vi "to string 1.0.vi"(8 "error in (no error)":errorcluster, 11 "Formatter Config in":refnum<class "csv-formatter Config.lvclass">) -> (0 "error out":errorcluster, 2 "data":string, 3 "Formatter Config out":refnum<class "csv-formatter Config.lvclass">)   [LabVIEW 2015, in "csv-formatter Config.lvclass"]
uses:
  csv-formatter Config.lvclass
  csv-formatter Config.lvclass/csv-formatter Config.ctl
  Result Config.ctl
  <vilib>/NI/Configuration Framework/serializable configuration/NISE_CEF_serializable configuration.lvclass
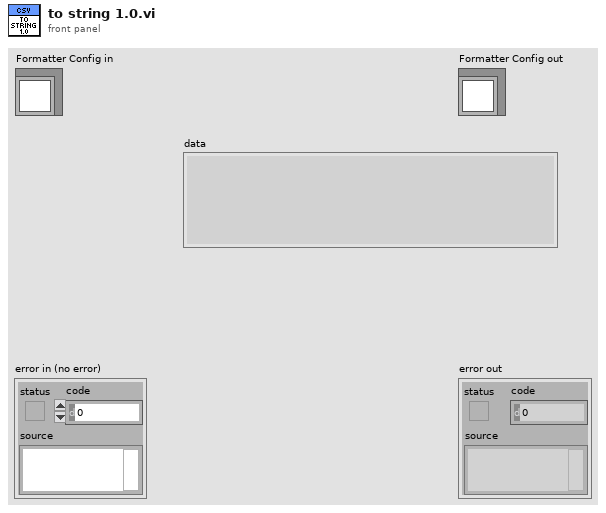
[diagram p1: front panel]
types:
  T1 = typedef "Result Config.ctl" = string[]
  T2 = typedef "Report Header Config.ctl" = string[][]
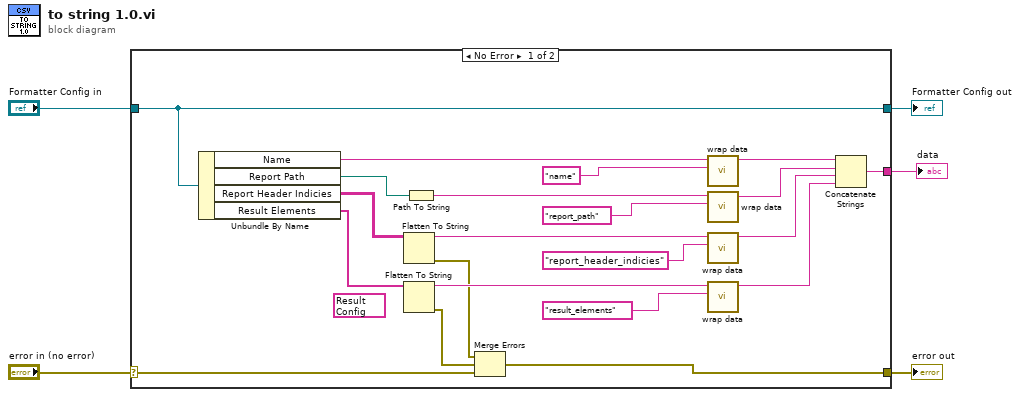
[diagram p0: block diagram]
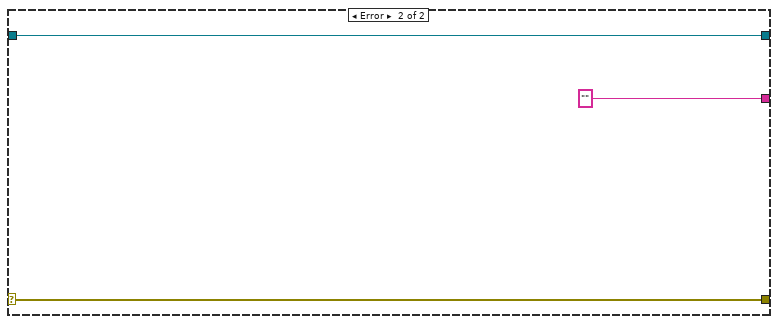
[diagram p2: hidden frame]
diagram:
  n1 = case shown="No Error" "error in (no error)" {
    selector: "error in (no error)" -> [w26 w29]
    tunnel: [w8 w29] -> w4
    tunnel: [w25 w28] -> w2
    tunnel: "Formatter Config in" -> [w25 w28]
    tunnel: [w19 ""] -> w1
    frame No Error {
      (unwired) T1 ["Step Name", "Step Class", "Low Limit", "Measurement", "High Limit", "Comparison", "Duration"] ("Result Elements")
      n2 = Unbundle By Name(w25) -> ("Name"=w23:string, "Report Path"=w22:path, "Report Header Indicies"=w16:T2, "Result Elements"=w12:T1)
      n3 = Flatten To String(anything=w16) -> (data string=w15:string, error out=w7:errorcluster)  [unwired: 3 in, 1 out]
      n4 = Flatten To String(anything=w12) -> (data string=w11:string, error out=w6:errorcluster)  [unwired: 3 in, 1 out]
      n5 = Path To String(path=w22) -> (string=w21:string)
      n6 = Merge Errors(w7, w6, w26) -> (w8:errorcluster)
      n7 = call <vilib>:"wrap data.vi"("identifier"="name", "data to wrap"=w23) -> ("wrapped data"=w18:string)  [unwired: 9 in]
      n8 = call <vilib>:"wrap data.vi"("identifier"="report_path", "data to wrap"=w21) -> ("wrapped data"=w17:string)  [unwired: 9 in]
      n9 = call <vilib>:"wrap data.vi"("identifier"="report_header_indicies", "data to wrap"=w15) -> ("wrapped data"=w13:string)  [unwired: 9 in]
      n10 = call <vilib>:"wrap data.vi"("identifier"="result_elements", "data to wrap"=w11) -> ("wrapped data"=w10:string)  [unwired: 9 in]
      n11 = Concatenate Strings(w18, w17, w13, w10) -> (w19:string)
    }
    frame Error {
    }
  }
  "error out" <- w4
  "Formatter Config out" <- w2
  "data" <- w1
